vi "Send Trigger Command.vi"(8 "error in (no error)":errorcluster, 9 "Trigger data":T1, 10 "Trigger Received in":T2, 11 "Trigger Event in":refnum<user-event>) -> (0 "error out":errorcluster, 3 "Trigger Event out":refnum<user-event>)   [LabVIEW 2012, in "Waveform Data Logger Engine.lvlib"]
uses:
  Waveform Data Logger Engine.lvlib
  Types/Trigger Received.ctl
  Types/Trigger Event Data.ctl
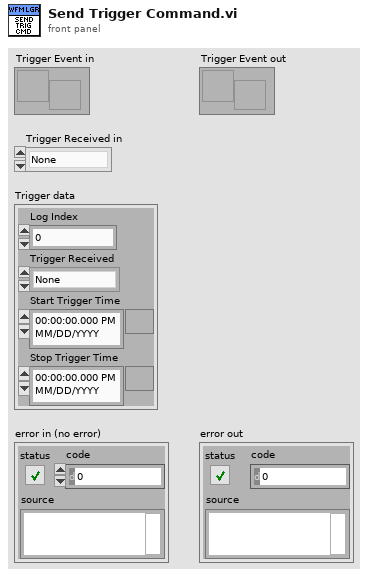
[diagram p1: front panel]
types:
  T1 = typedef "Waveform Data Logger Engine.lvlib/Trigger Event Data.ctl" = cluster{"Log Index":i32, "Trigger Received":T2, "Start Trigger Time":timestamp, "Stop Trigger Time":timestamp}
  T2 = typedef "Waveform Data Logger Engine.lvlib/Trigger Received.ctl" = enum16{"None", "Start", "Stop", "Both", "Disable"}
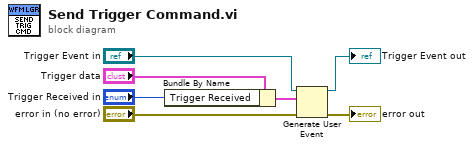
[diagram p0: block diagram]
diagram:
  n1 = Bundle By Name(cluster="Trigger data", "Trigger Received"="Trigger Received in") -> (w3:T1)
  n2 = Generate User Event(user event="Trigger Event in", event data cluster=w3, error in="error in (no error)") -> (user event out=→"Trigger Event out":refnum<user-event>, error out=→"error out":errorcluster)
